vi "Packet to List.vi"(1 "Packet":string) -> (0 "List":string[](array[string]))   [LabVIEW 2021, in "d13.lvlib"]
uses:
  d13.lvlib
  <vilib>/regexp/Match Regular Expression.xnode
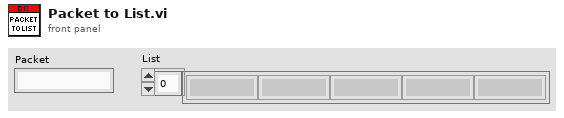
[diagram p1: front panel]
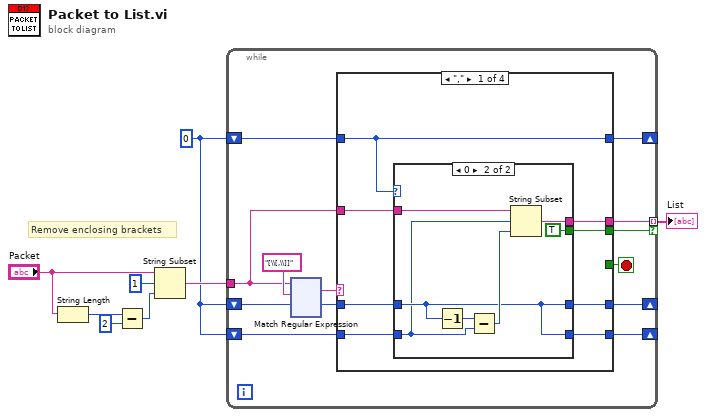
[diagram p0: block diagram]
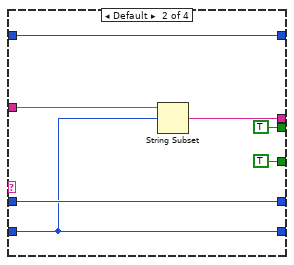
[diagram p3: hidden frame]
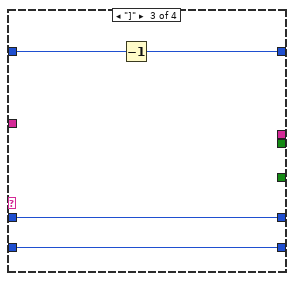
[diagram p4: hidden frame]
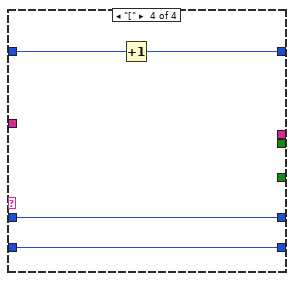
[diagram p5: hidden frame]
diagram:
  w2 = 0
  # "Remove enclosing brackets"
  n1 = String Length(string="Packet") -> (length=w5:i32)
  n2 = Subtract(x=w5, y=2) -> (x-y=w4:i32)
  n3 = String Subset(string="Packet", offset (0)=1, length (rest)=w4) -> (substring=w8:string)
  n4 = while {
    shift-right: [w19] -> _
    shift-left: w2 -> [w20]
    shift-right: [w9] -> _
    shift-left: w2 -> [w18]
    tunnel: w8 -> [w17]
    shift-right: [w13] -> _
    shift-left: w2 -> [w14]
    tunnel: [w16] -> w1 mode=indexing if=w15
    stop <- w10 stop-if-true
    n5 = xnode "Match Regular Expression"("input string"=w17, "regular expression"="[\\[,\\]]", "offset (0)"=w18) -> ("whole match"=w11:string, "offset past match"=w12:i32)  [unwired: 3 in, 3 out]
    n6 = case shown="\",\"" w11 {
      tunnel: w20 -> [w22 w45 w49 w53]
      tunnel: [w22 w45 w48 w52] -> w19
      tunnel: w12 -> [w28 w41 w47 w51]
      tunnel: w17 -> [w29 w42 _ _]
      tunnel: w14 -> [w25 w40 w46 w50]
      tunnel: [w27 w39 _ _] -> w16
      tunnel: [w26 TRUE _ _] -> w15
      tunnel: [w24 w40 w46 w50] -> w13
      tunnel: [_ TRUE _ _] -> w10
      tunnel: [w23 w41 w47 w51] -> w9
      frame "," {
        n7 = case shown="0" w22 {
          tunnel: w29 -> [_ w38]
          tunnel: w28 -> [w31 w33]
          tunnel: [_ w37] -> w27
          tunnel: w25 -> [w30 w32]
          tunnel: [_ TRUE] -> w26
          tunnel: [w30 w33] -> w24
          tunnel: [w31 w33] -> w23
          frame Default {
          }
          frame 0 {
            n8 = Decrement(x=w33) -> (x-1=w35:i32)
            n9 = Subtract(x=w35, y=w32) -> (x-y=w36:i32)
            n10 = String Subset(string=w38, offset (0)=w32, length (rest)=w36) -> (substring=w37:string)
          }
        }
      }
      frame Default {
        n11 = String Subset(string=w42, offset (0)=w40) -> (substring=w39:string)  [unwired: 1 in]
      }
      frame "]" {
        n12 = Decrement(x=w49) -> (x-1=w48:i32)
      }
      frame "[" {
        n13 = Increment(x=w53) -> (x+1=w52:i32)
      }
    }
  }
  "List" <- w1
